vi "ClearBoard Loop test.vi"() -> ()   [LabVIEW 2020]
uses:
  controls/keyboard 3x3.ctl
  controls/Player.ctl
  <vilib>/ErrorRing/Error Ring.xnode
panel:
  out "time parallelized loop (ms)":dbl
  out "time non parallelized loop (ms)":dbl
  in  "Gameboard":T1
  # "for me it was 2.232 ms for loop without parallelism enabled\nand 2.383 ms with"
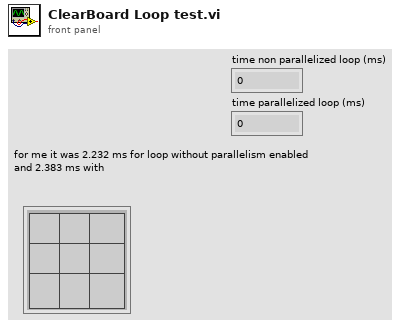
[diagram p1: front panel]
types:
  T1 = typedef "keyboard 3x3.ctl" = cluster{"Button 1":bool, "Button 2":bool, "Button 3":bool, "Button 4":bool, "Button 5":bool, "Button 6":bool, "Button 7":bool, "Button 8":bool, "Button 9":bool}
  T2 = typedef "Player.ctl" = enum16{"None", "Player 1", "Player 2"}
  T3 = enum8{"Enabled", "Disabled", "Disabled and Grayed Out"}
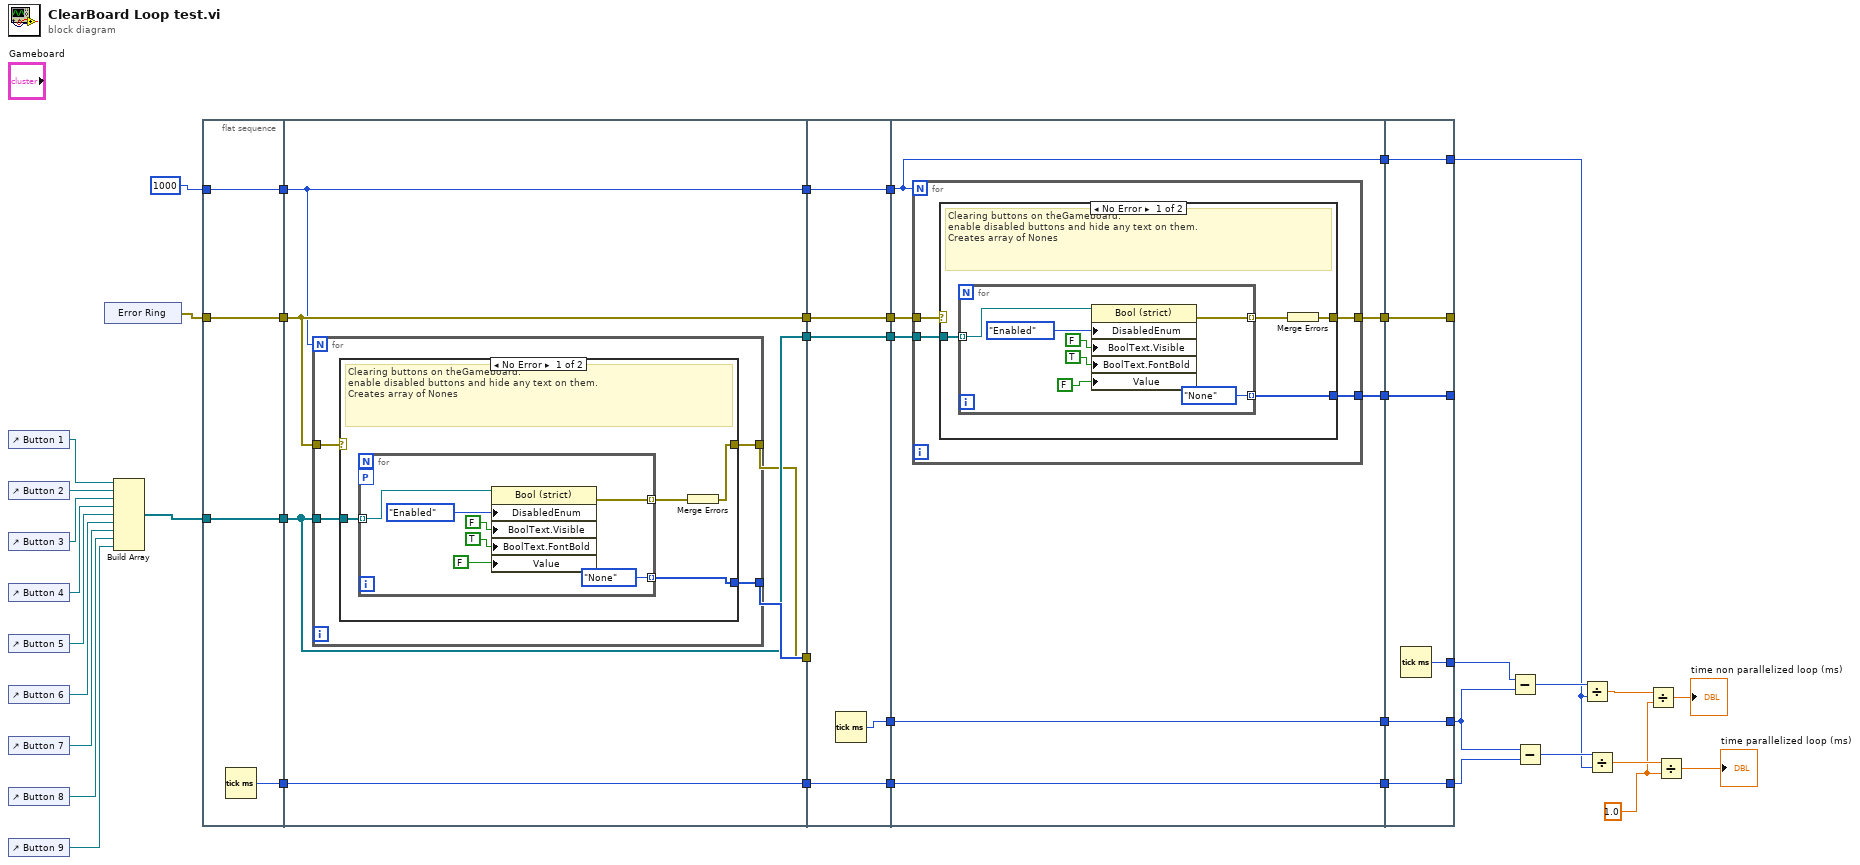
[diagram p0: block diagram]
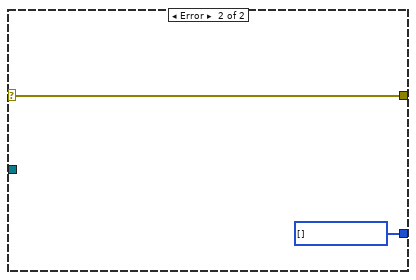
[diagram p2: hidden frame]
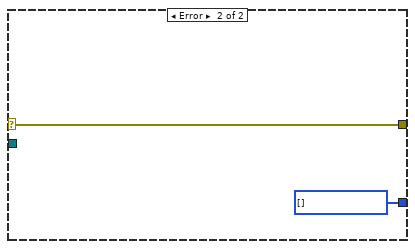
[diagram p3: hidden frame]
diagram:
  w3 = 1.0 ("y")
  n1 = control-ref of="Button 1"() -> (w43:refnum<vi>)
  n2 = control-ref of="Button 2"() -> (w42:refnum<vi>)
  n3 = control-ref of="Button 3"() -> (w41:refnum<vi>)
  n4 = control-ref of="Button 4"() -> (w40:refnum<vi>)
  n5 = control-ref of="Button 5"() -> (w39:refnum<vi>)
  n6 = control-ref of="Button 6"() -> (w38:refnum<vi>)
  n7 = control-ref of="Button 7"() -> (w37:refnum<vi>)
  n8 = control-ref of="Button 8"() -> (w36:refnum<vi>)
  n9 = control-ref of="Button 9"() -> (w35:refnum<vi>)
  n10 = xnode "Error Ring"() -> ("error out"=w29:errorcluster)
  n11 = Build Array(w43, w42, w41, w40, w39, w38, w37, w36, w35) -> (w33:refnum<vi>[])
  n12 = flat-sequence {
    tunnel: w33 -> [w47]
    tunnel: [w47] -> w32
    tunnel: w29 -> [w46]
    tunnel: [w46] -> w28
    tunnel: [w45] -> w27
    tunnel: 1000 -> [w45]
    tunnel: [w44] -> w16
    tunnel: [w53] -> w34
    tunnel: w32 -> [w52]
    tunnel: [w52] -> w31
    tunnel: w28 -> [w51]
    tunnel: w27 -> [w50]
    tunnel: [w51] -> w24
    tunnel: [w50] -> w22
    tunnel: [w49] -> w21
    tunnel: [w48] -> w17
    tunnel: w16 -> [w48]
    tunnel: w34 -> [_]
    tunnel: w31 -> [w75]
    tunnel: [w75] -> w30
    tunnel: [w74] -> w25
    tunnel: w24 -> [w74]
    tunnel: [w73] -> w23
    tunnel: w22 -> [w73]
    tunnel: w21 -> [_]
    tunnel: [w72] -> w18
    tunnel: w17 -> [w72]
    tunnel: [w71] -> w14
    tunnel: w30 -> [w82]
    tunnel: w25 -> [w81]
    tunnel: w23 -> [w76]
    tunnel: [w80] -> w20
    tunnel: [w79] -> w19
    tunnel: w18 -> [w77]
    tunnel: [w78] -> w15
    tunnel: w14 -> [w78]
    tunnel: [w77] -> w13
    tunnel: [w76] -> w5
    tunnel: [w104] -> _
    tunnel: [w105] -> _
    tunnel: w20 -> [w105]
    tunnel: w19 -> [w104]
    tunnel: w15 -> [w101]
    tunnel: [w103] -> w12
    tunnel: [w102] -> w11
    tunnel: w13 -> [w102]
    tunnel: [w101] -> w10
    tunnel: w5 -> [w100]
    tunnel: [w100] -> w4
    frame #0 {
      n13 = Tick Count (ms)() -> (millisecond timer value=w44:u32)
    }
    frame #1 {
      n14 = for {
        N: w50 -> [_]
        tunnel: [w57] -> w53
        tunnel: w52 -> [w56]
        tunnel: w51 -> [w55]
        tunnel: [w54] -> w49
        n15 = case shown="No Error" w55 {
          selector: w55 -> [_ w70]
          tunnel: w56 -> [w61 _]
          tunnel: [w59 w70] -> w54
          tunnel: [w58 w69] -> w57
          frame No Error {
            # "Clearing buttons on theGameboard: \nenable disabled buttons and hide any text on them.\nCreates array of Nones"
            n16 = for {
              tunnel: w61 -> [w68] mode=indexing
              workers-P: _ -> [_]
              tunnel: [w65] -> w60 mode=indexing
              tunnel: [Player."None" ("Player")] -> w58 mode=indexing
              n17 = property class="Bool (strict)"(reference=w68, "DisabledEnum"=T3."Enabled" ("Disabled"), "BoolText.Visible"=FALSE ("Boolean Text.Visible"), "BoolText.FontBold"=TRUE ("Boolean Text.Font:Bold"), "Value"=FALSE) -> (error out=w65:errorcluster)  [unwired: 1 in, 1 out]
            }
            n18 = Merge Errors(w60) -> (w59:errorcluster)
          }
          frame Error {
            w69 = T2[] [] items=["None", "Player 1", "Player 2"]
          }
        }
      }
    }
    frame #2 {
      n19 = Tick Count (ms)() -> (millisecond timer value=w71:u32)
    }
    frame #3 {
      n20 = for {
        N: w76 -> [_]
        tunnel: w82 -> [w86]
        tunnel: w81 -> [w85]
        tunnel: [w84] -> w80
        tunnel: [w83] -> w79
        n21 = case shown="No Error" w85 {
          selector: w85 -> [_ w99]
          tunnel: w86 -> [w90 _]
          tunnel: [w88 w99] -> w83
          tunnel: [w87 w98] -> w84
          frame No Error {
            # "Clearing buttons on theGameboard: \nenable disabled buttons and hide any text on them.\nCreates array of Nones"
            n22 = for {
              tunnel: w90 -> [w97] mode=indexing
              tunnel: [w94] -> w89 mode=indexing
              tunnel: [Player."None" ("Player")] -> w87 mode=indexing
              n23 = property class="Bool (strict)"(reference=w97, "DisabledEnum"=T3."Enabled" ("Disabled"), "BoolText.Visible"=FALSE ("Boolean Text.Visible"), "BoolText.FontBold"=TRUE ("Boolean Text.Font:Bold"), "Value"=FALSE) -> (error out=w94:errorcluster)  [unwired: 1 in, 1 out]
            }
            n24 = Merge Errors(w89) -> (w88:errorcluster)
          }
          frame Error {
            w98 = T2[] [] items=["None", "Player 1", "Player 2"]
          }
        }
      }
    }
    frame #4 {
      n25 = Tick Count (ms)() -> (millisecond timer value=w103:u32)
    }
  }
  n26 = Subtract(x=w12, y=w10) -> (x-y=w9:u32)
  n27 = Subtract(x=w10, y=w11) -> (x-y=w7:u32)
  n28 = Divide(x=w9, y=w4) -> (x/y=w8:dbl)
  n29 = Divide(x=w7, y=w4) -> (x/y=w6:dbl)
  n30 = Divide(x=w8, y=w3) -> (x/y=→"time non parallelized loop (ms)":dbl)
  n31 = Divide(x=w6, y=w3) -> (x/y=→"time parallelized loop (ms)":dbl)
